vi "SBML_Reactions_Parser.vi"(6 "error in (no error)":errorcluster, 9 "Input SBML File":string) -> (0 "error out":errorcluster, 1 "Reaction Math":string[][](table), 2 "Reaction Info":string[][](table), 3 "Reac_cnt":i32)   [LabVIEW 2014]
doc: "This VI extract the information of reactions present in SBML file. It takes the complete SBML file as input, and outputs: \nReac_Cnt --> How many reactions are there\nReac_Id_Arr --> Array of reactions\nReac_rev_Arr --> Indicates if the corresponding indexed reaction is reversible\nReac_fast --> Indicates if the corresponding indexed reaction is fast\nKinetic Laws --> Extract the list of kinetic laws of each reaction\nModifiers_Arr --> Array of modifiers (or catalysts)\nProducts_Arr --> Array of products of reactions\n\nDesigned by HB\nhaba@dtu.dk"
panel:
  out "P-Const":string[](array[string])
  out "Mod Cnt":string[](array[string])
  out "Prod Cnt":string[](array[string])
  out "Reac Cnt":string[](array[string])
  out "R-Const":string[](array[string])
  out "Compartment":string[](array[string])
  out "Name":string[](array[string])
  out "P-Stoich_Arr":string[](array[string])
  out "R-Stoich":string[](array[string])
  out "LP_Values":string[](array[string])
  out "Local Param":string[](array[string])
  out "LP Cnt":string[](array[string])
  out "Math":string[](array[string])
  out "Modifiers":string[](array[string])
  out "Products":string[](array[string])
  out "Reactants":string[](array[string])
  out "Fast":string[](array[string])
  out "Reversible":string[](array[string])
  out "ID":string[](array[string])
  out "List of Reactions":string
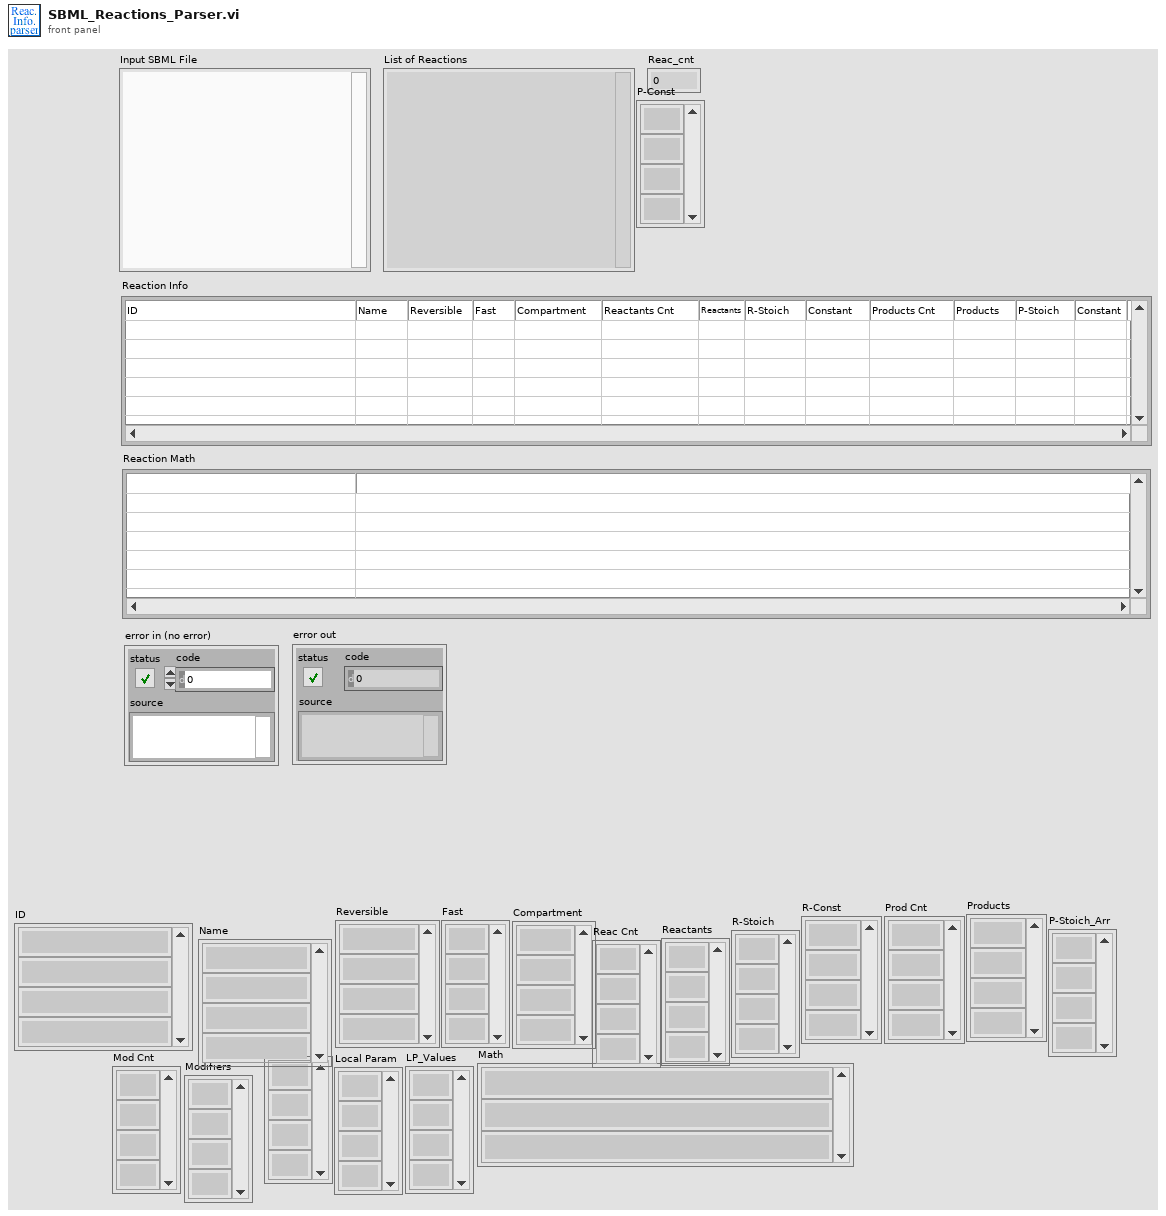
[diagram p1: front panel]
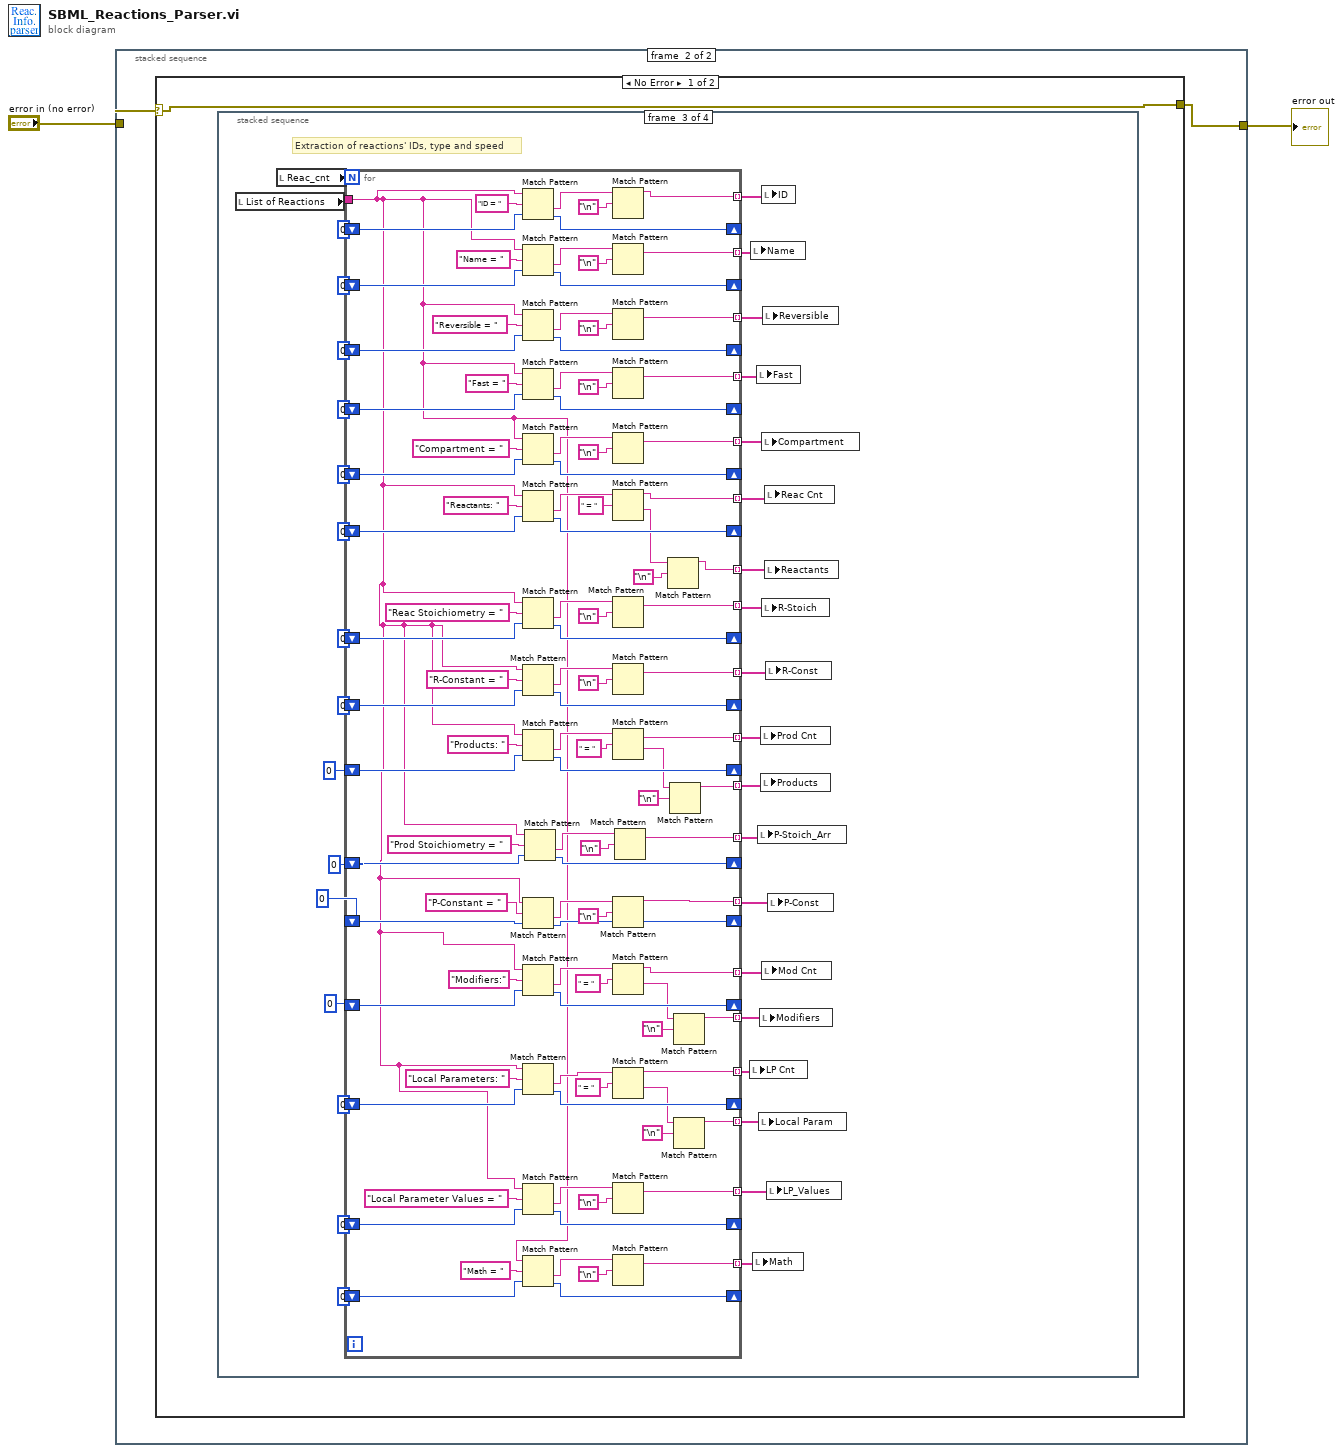
[diagram p0: block diagram]
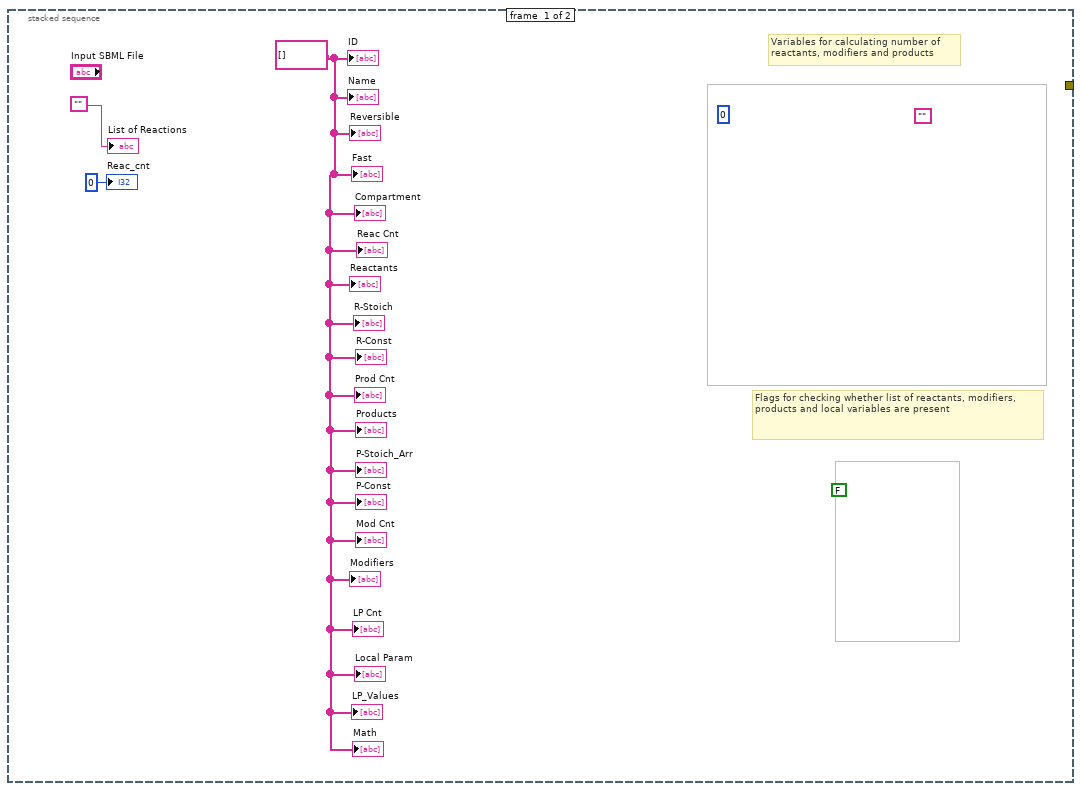
[diagram p2: hidden frame]
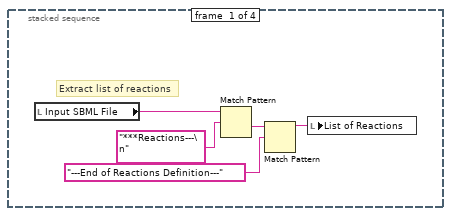
[diagram p3: hidden frame]
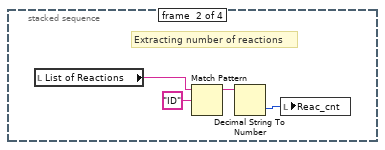
[diagram p4: hidden frame]
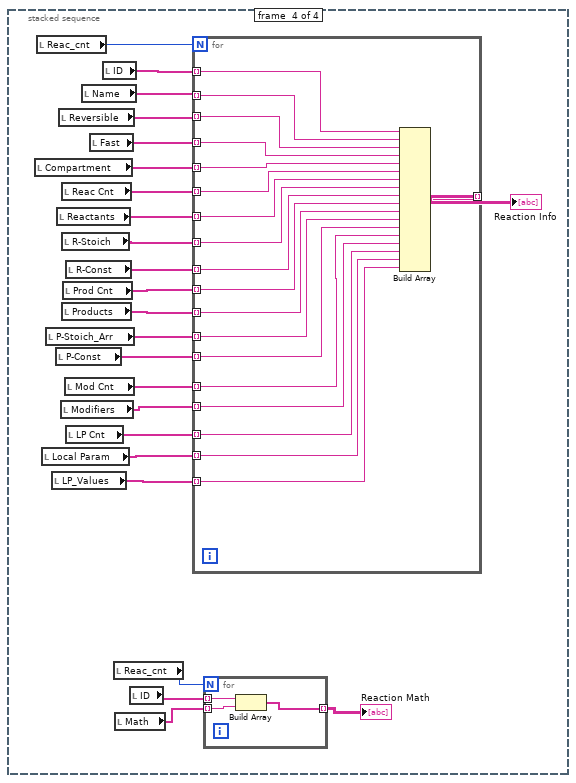
[diagram p5: hidden frame]
diagram:
  n1 = stacked-sequence {
    tunnel: "error in (no error)" -> [_ w6]
    tunnel: [_ w7] -> w1
    frame #0 {
      w3 = string[] [] ("Sp_Id_Arr")
      (unwired) FALSE ("R-lst")
      (unwired) "" ("Full SBML File")
      (unwired) 0 ("Rctns_Indx")
      # "Flags for checking whether list of reactants, modifiers, products and local variables are present"
      # "Variables for calculating number of \nreactants, modifiers and products"
      "List of Reactions" <- "" ("Full SBML File")
      "Reac_cnt" <- 0 ("Reac_cnt")
      "ID" <- w3
      "Reversible" <- w3
      "Fast" <- w3
      "Reactants" <- w3
      "Products" <- w3
      "Modifiers" <- w3
      "Math" <- w3
      "LP Cnt" <- w3
      "LP_Values" <- w3
      "Local Param" <- w3
      "R-Stoich" <- w3
      "P-Stoich_Arr" <- w3
      "Name" <- w3
      "Compartment" <- w3
      "R-Const" <- w3
      "Reac Cnt" <- w3
      "Prod Cnt" <- w3
      "Mod Cnt" <- w3
      "P-Const" <- w3
    }
    frame #1 {
      n2 = case shown="No Error" w6 {
        selector: w6 -> [w8 w203]
        tunnel: [w8 w203] -> w7
        frame No Error {
          n3 = stacked-sequence {
            frame #0 {
              # "Extract list of reactions"
              n4 = local read "Input SBML File"() -> (w12:string)
              n5 = Match Pattern(string=w12, regular expression="***Reactions---\n") -> (after substring=w10:string)  [unwired: 1 in, 3 out]
              n6 = Match Pattern(string=w10, regular expression="---End of Reactions Definition---") -> (before substring=w13:string)  [unwired: 1 in, 3 out]
              n7 = local write "List of Reactions"(w13) -> ()
            }
            frame #1 {
              # "Extracting number of reactions"
              n8 = local read "List of Reactions"() -> (w14:string)
              n9 = Match Pattern(string=w14, regular expression="ID") -> (before substring=w17:string)  [unwired: 1 in, 3 out]
              n10 = Decimal String To Number(string=w17) -> (number=w15:i32)  [unwired: 2 in, 1 out]
              n11 = local write "Reac_cnt"(w15) -> ()
            }
            frame #2 {
              # "Extraction of reactions' IDs, type and speed"
              n12 = local read "List of Reactions"() -> (w52:string)
              n13 = local read "Reac_cnt"() -> (w51:i32)
              n14 = for {
                N: w51 -> [_]
                tunnel: w52 -> [w54]
                tunnel: [w153] -> w53 mode=indexing
                shift-right: [w151] -> _
                shift-left: 0 ("offset of match") -> [w152]
                tunnel: [w148] -> w48 mode=indexing
                shift-right: [w150] -> _
                shift-left: 0 ("offset of match") -> [w149]
                tunnel: [w141] -> w47 mode=indexing
                shift-right: [w139] -> _
                shift-left: 0 ("offset of match") -> [w140]
                tunnel: [w129] -> w43 mode=indexing
                shift-right: [w127] -> _
                shift-left: 0 ("offset of match") -> [w128]
                tunnel: [w136] -> w44 mode=indexing
                shift-right: [w138] -> _
                shift-left: 0 ("offset of match") -> [w137]
                tunnel: [w124] -> w40 mode=indexing
                shift-right: [w126] -> _
                shift-left: 0 ("offset of match") -> [w125]
                tunnel: [w118] -> w24 mode=indexing
                shift-right: [w116] -> _
                shift-left: 0 ("offset of match") -> [w117]
                tunnel: [w89] -> w29 mode=indexing
                shift-right: [w87] -> _
                shift-left: 0 ("offset of match") -> [w88]
                tunnel: [w95] -> w30 mode=indexing
                shift-right: [w97] -> _
                shift-left: 0 ("offset of match") -> [w96]
                tunnel: [w106] -> w34 mode=indexing
                tunnel: [w100] -> w33 mode=indexing
                shift-right: [w98] -> _
                shift-left: 0 ("offset of match") -> [w99]
                tunnel: [w64] -> w36 mode=indexing
                shift-right: [w107] -> _
                shift-left: 0 ("offset of match") -> [w108]
                tunnel: [w113] -> w37 mode=indexing
                shift-right: [w115] -> _
                shift-left: 0 ("offset of match") -> [w114]
                tunnel: [w83] -> w27 mode=indexing
                shift-right: [w81] -> _
                shift-left: 0 ("offset of match") -> [w82]
                tunnel: [w80] -> w25 mode=indexing
                tunnel: [w73] -> w23 mode=indexing
                tunnel: [w69] -> w22 mode=indexing
                tunnel: [w63] -> w21 mode=indexing
                tunnel: [w60] -> w18 mode=indexing
                shift-right: [w62] -> _
                shift-left: 0 ("offset of match") -> [w61]
                shift-right: [w55] -> _
                shift-left: 0 ("offset of match") -> [w56]
                n15 = Match Pattern(string=w54, regular expression="ID = ", offset (0)=w152) -> (after substring=w154:string, offset past match=w151:i32)  [unwired: 2 out]
                n16 = Match Pattern(string=w54, regular expression="Name = ", offset (0)=w149) -> (after substring=w147:string, offset past match=w150:i32)  [unwired: 2 out]
                n17 = Match Pattern(string=w54, regular expression="Reversible = ", offset (0)=w140) -> (after substring=w142:string, offset past match=w139:i32)  [unwired: 2 out]
                n18 = Match Pattern(string=w54, regular expression="Fast = ", offset (0)=w128) -> (after substring=w130:string, offset past match=w127:i32)  [unwired: 2 out]
                n19 = Match Pattern(string=w54, regular expression="Compartment = ", offset (0)=w137) -> (after substring=w135:string, offset past match=w138:i32)  [unwired: 2 out]
                n20 = Match Pattern(string=w54, regular expression="Reactants: ", offset (0)=w125) -> (after substring=w123:string, offset past match=w126:i32)  [unwired: 2 out]
                n21 = Match Pattern(string=w54, regular expression="Reac Stoichiometry = ", offset (0)=w117) -> (after substring=w119:string, offset past match=w116:i32)  [unwired: 2 out]
                n22 = Match Pattern(string=w54, regular expression="R-Constant = ", offset (0)=w88) -> (after substring=w90:string, offset past match=w87:i32)  [unwired: 2 out]
                n23 = Match Pattern(string=w54, regular expression="Products: ", offset (0)=w96) -> (after substring=w94:string, offset past match=w97:i32)  [unwired: 2 out]
                n24 = Match Pattern(string=w54, regular expression="P-Constant = ", offset (0)=w61) -> (after substring=w59:string, offset past match=w62:i32)  [unwired: 2 out]
                n25 = Match Pattern(string=w54, regular expression="Modifiers:", offset (0)=w99) -> (after substring=w101:string, offset past match=w98:i32)  [unwired: 2 out]
                n26 = Match Pattern(string=w54, regular expression="Local Parameters: ", offset (0)=w108) -> (after substring=w65:string, offset past match=w107:i32)  [unwired: 2 out]
                n27 = Match Pattern(string=w54, regular expression="Local Parameter Values = ", offset (0)=w114) -> (after substring=w112:string, offset past match=w115:i32)  [unwired: 2 out]
                n28 = Match Pattern(string=w54, regular expression="Math = ", offset (0)=w82) -> (after substring=w84:string, offset past match=w81:i32)  [unwired: 2 out]
                n29 = Match Pattern(string=w54, regular expression="Prod Stoichiometry = ", offset (0)=w56) -> (after substring=w105:string, offset past match=w55:i32)  [unwired: 2 out]
                n30 = Match Pattern(string=w154, regular expression="\n") -> (before substring=w153:string)  [unwired: 1 in, 3 out]
                n31 = Match Pattern(string=w147, regular expression="\n") -> (before substring=w148:string)  [unwired: 1 in, 3 out]
                n32 = Match Pattern(string=w142, regular expression="\n") -> (before substring=w141:string)  [unwired: 1 in, 3 out]
                n33 = Match Pattern(string=w130, regular expression="\n") -> (before substring=w129:string)  [unwired: 1 in, 3 out]
                n34 = Match Pattern(string=w135, regular expression="\n") -> (before substring=w136:string)  [unwired: 1 in, 3 out]
                n35 = Match Pattern(string=w123, regular expression=" = ") -> (before substring=w124:string, after substring=w77:string)  [unwired: 1 in, 2 out]
                n36 = Match Pattern(string=w119, regular expression="\n") -> (before substring=w118:string)  [unwired: 1 in, 3 out]
                n37 = Match Pattern(string=w90, regular expression="\n") -> (before substring=w89:string)  [unwired: 1 in, 3 out]
                n38 = Match Pattern(string=w94, regular expression=" = ") -> (before substring=w95:string, after substring=w74:string)  [unwired: 1 in, 2 out]
                n39 = Match Pattern(string=w59, regular expression="\n") -> (before substring=w60:string)  [unwired: 1 in, 3 out]
                n40 = Match Pattern(string=w101, regular expression=" = ") -> (before substring=w100:string, after substring=w70:string)  [unwired: 1 in, 2 out]
                n41 = Match Pattern(string=w65, regular expression=" = ") -> (before substring=w64:string, after substring=w68:string)  [unwired: 1 in, 2 out]
                n42 = Match Pattern(string=w112, regular expression="\n") -> (before substring=w113:string)  [unwired: 1 in, 3 out]
                n43 = Match Pattern(string=w84, regular expression="\n") -> (before substring=w83:string)  [unwired: 1 in, 3 out]
                n44 = Match Pattern(string=w105, regular expression="\n") -> (before substring=w106:string)  [unwired: 1 in, 3 out]
                n45 = Match Pattern(string=w77, regular expression="\n") -> (before substring=w80:string)  [unwired: 1 in, 3 out]
                n46 = Match Pattern(string=w74, regular expression="\n") -> (before substring=w73:string)  [unwired: 1 in, 3 out]
                n47 = Match Pattern(string=w70, regular expression="\n") -> (before substring=w69:string)  [unwired: 1 in, 3 out]
                n48 = Match Pattern(string=w68, regular expression="\n") -> (before substring=w63:string)  [unwired: 1 in, 3 out]
              }
              n49 = local write "LP Cnt"(w36) -> ()
              n50 = local write "Name"(w48) -> ()
              n51 = local write "Math"(w27) -> ()
              n52 = local write "Fast"(w43) -> ()
              n53 = local write "P-Stoich_Arr"(w34) -> ()
              n54 = local write "Local Param"(w21) -> ()
              n55 = local write "Modifiers"(w22) -> ()
              n56 = local write "Prod Cnt"(w30) -> ()
              n57 = local write "Products"(w23) -> ()
              n58 = local write "ID"(w53) -> ()
              n59 = local write "Compartment"(w44) -> ()
              n60 = local write "R-Stoich"(w24) -> ()
              n61 = local write "Mod Cnt"(w33) -> ()
              n62 = local write "Reversible"(w47) -> ()
              n63 = local write "Reac Cnt"(w40) -> ()
              n64 = local write "Reactants"(w25) -> ()
              n65 = local write "R-Const"(w29) -> ()
              n66 = local write "LP_Values"(w37) -> ()
              n67 = local write "P-Const"(w18) -> ()
            }
            frame #3 {
              n68 = local read "Compartment"() -> (w175:string[])
              n69 = local read "Reac_cnt"() -> (w180:i32)
              n70 = local read "Local Param"() -> (w163:string[])
              n71 = local read "P-Stoich_Arr"() -> (w167:string[])
              n72 = local read "LP_Values"() -> (w162:string[])
              n73 = local read "P-Const"() -> (w157:string[])
              n74 = local read "Reactants"() -> (w173:string[])
              n75 = local read "Reversible"() -> (w177:string[])
              n76 = local read "Modifiers"() -> (w165:string[])
              n77 = local read "Reac Cnt"() -> (w174:string[])
              n78 = local read "R-Stoich"() -> (w170:string[])
              n79 = local read "Products"() -> (w168:string[])
              n80 = local read "Prod Cnt"() -> (w169:string[])
              n81 = local read "Mod Cnt"() -> (w166:string[])
              n82 = local read "R-Const"() -> (w172:string[])
              n83 = local read "LP Cnt"() -> (w164:string[])
              n84 = local read "Name"() -> (w178:string[])
              n85 = local read "Fast"() -> (w176:string[])
              n86 = local read "ID"() -> (w179:string[])
              n87 = local read "Reac_cnt"() -> (w171:i32)
              n88 = local read "Math"() -> (w160:string[])
              n89 = local read "ID"() -> (w161:string[])
              n90 = for {
                N: w180 -> [_]
                tunnel: w179 -> [w202] mode=indexing
                tunnel: w178 -> [w201] mode=indexing
                tunnel: w177 -> [w200] mode=indexing
                tunnel: w176 -> [w199] mode=indexing
                tunnel: w175 -> [w198] mode=indexing
                tunnel: w174 -> [w197] mode=indexing
                tunnel: w173 -> [w196] mode=indexing
                tunnel: w170 -> [w195] mode=indexing
                tunnel: w172 -> [w194] mode=indexing
                tunnel: [w193] -> w159 mode=indexing
                tunnel: w169 -> [w192] mode=indexing
                tunnel: w168 -> [w191] mode=indexing
                tunnel: w167 -> [w190] mode=indexing
                tunnel: w166 -> [w189] mode=indexing
                tunnel: w165 -> [w188] mode=indexing
                tunnel: w164 -> [w187] mode=indexing
                tunnel: w163 -> [w186] mode=indexing
                tunnel: w162 -> [w185] mode=indexing
                tunnel: w157 -> [w184] mode=indexing
                n91 = Build Array(w202, w201, w200, w199, w198, w197, w196, w195, w194, w192, w191, w190, w184, w189, w188, w187, w186, w185) -> (w193:string[])
              }
              "Reaction Info" <- w159
              n92 = for {
                N: w171 -> [_]
                tunnel: [w183] -> w158 mode=indexing
                tunnel: w161 -> [w182] mode=indexing
                tunnel: w160 -> [w181] mode=indexing
                n93 = Build Array(w182, w181) -> (w183:string[])
              }
              "Reaction Math" <- w158
            }
          }
        }
        frame Error {
        }
      }
    }
  }
  "error out" <- w1
